vi "LVClass_WavefrontCorrectorSet Get Parameter Int Limits.vi"(0 "WavefrontCorrectorSet in":refnum<class "WavefrontCorrectorSet.lvclass">, 5 "parameter_name":string, 11 "error in (no error)":errorcluster) -> (4 "WavefrontCorrectorSet out":refnum<class "WavefrontCorrectorSet.lvclass">, 6 "min":i32, 8 "max":i32, 15 "error out":errorcluster)   [LabVIEW 2020, in "WavefrontCorrectorSet.lvclass"]
doc: "WavefrontCorrectorSet parameter range getter for parameter of type integer.\n\n--------------------------------------------------------------------------------\n\n<B>wavefrontcorrector_setIn </B> : WavefrontCorrectorSet object.\n<B>wavefrontcorrector_setOut </B> : WavefrontCorrectorSet object.\n<B>parameter_name </B> : Parameter name.\n<B>min </B> : Minimum value accepted.\n<B>max </B> : Maximum value accepted.\n<B>ErrorIn </B> : Error\n<B>ErrorOut </B> : Error\n\n--------------------------------------------------------------------------------"
uses:
  WavefrontCorrectorSet.lvclass
  WavefrontCorrectorSet.lvclass/WavefrontCorrectorSet.ctl
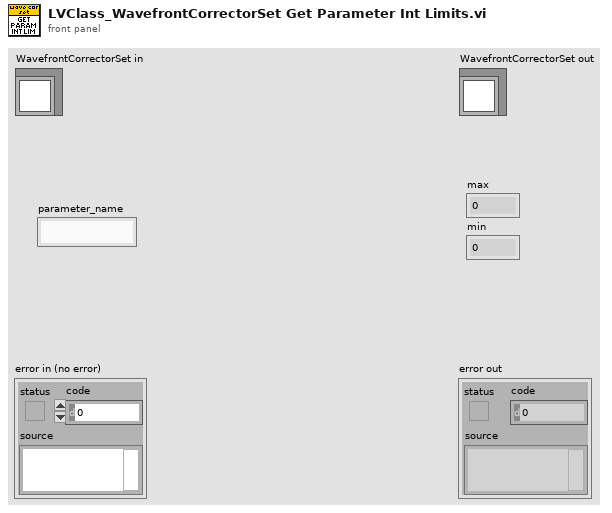
[diagram p1: front panel]
types:
  T1 = typedef "ClassID.ctl" = i64
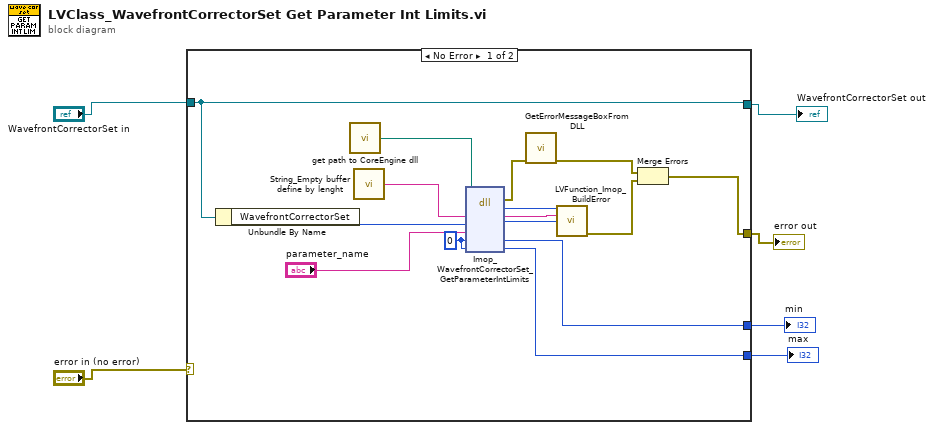
[diagram p0: block diagram]
diagram:
  n1 = case shown="No Error" "error in (no error)" {
    selector: "error in (no error)" -> [_ w22]
    tunnel: "WavefrontCorrectorSet in" -> [w14 w23]
    tunnel: [w14 w23] -> w1
    tunnel: [w10 w22] -> w2
    tunnel: [w9 _] -> w6
    tunnel: [w8 _] -> w5
    frame No Error {
      w15 = 0 ("min")
      n2 = Unbundle By Name(w14) -> ("WavefrontCorrectorSet"=w13:T1)
      n3 = call "get path to CoreEngine dll.vi"() -> ("path to wavekit library"=w17:path)  [unwired: 14 in, 1 out]
      n4 = call "String_Empty buffer define by lenght.vi"() -> ("Empty buffer"=w19:string)  [unwired: 1 in]
      n5 = dll-call lib="D:/soft/HASO_v3/C_interface/Sources/Build/vc100/Release/c_interface_vc100.dll" fn="Imop_WavefrontCorrectorSet_GetParameterIntLimits"(path in=w17, "message"=w19, "objet"=w13, "parameter_name"="parameter_name", "min"=w15, "max"=w15) -> (error out=w16:errorcluster, "return type"=w21:i32, "message"=w20:string, "objet"=w7:i64, "min"=w9:i32, "max"=w8:i32)  [unwired: 3 in, 1 out]
      n6 = call "GetErrorMessageBoxFromDLL.vi"("error IN"=w16) -> ("error OUT"=w11:errorcluster)  [unwired: 10 in]
      n7 = call "LVFunction_Imop_BuildError.vi"("code"=w21, "String to Prepend to source (\"\")"=w20, "Adresse"=w7) -> ("error out"=w12:errorcluster)  [unwired: 12 in]
      n8 = Merge Errors(w11, w12) -> (w10:errorcluster)
    }
    frame Error {
    }
  }
  "error out" <- w2
  "WavefrontCorrectorSet out" <- w1
  "min" <- w6
  "max" <- w5
